vi "printScreen.vi"(8 "错误输出":errorcluster, 10 "记录时间":string, 11 "地址":refnum<visa-resource-name>) -> (0 "error out":errorcluster, 1 "图片路径":string, 3 "二维图片":picture)   [LabVIEW 2014]
panel:
  in  "路径":path=path "C:/image"
  in  "User name":string="anonymous"
  in  "Password":string="\n"
  out "standard output":string
  out "standard error":string
  in  "run minimized? (F)":bool=TRUE
  in  "path to BMP file":path=path "C:/image/gwt.png" caption="文件路径"
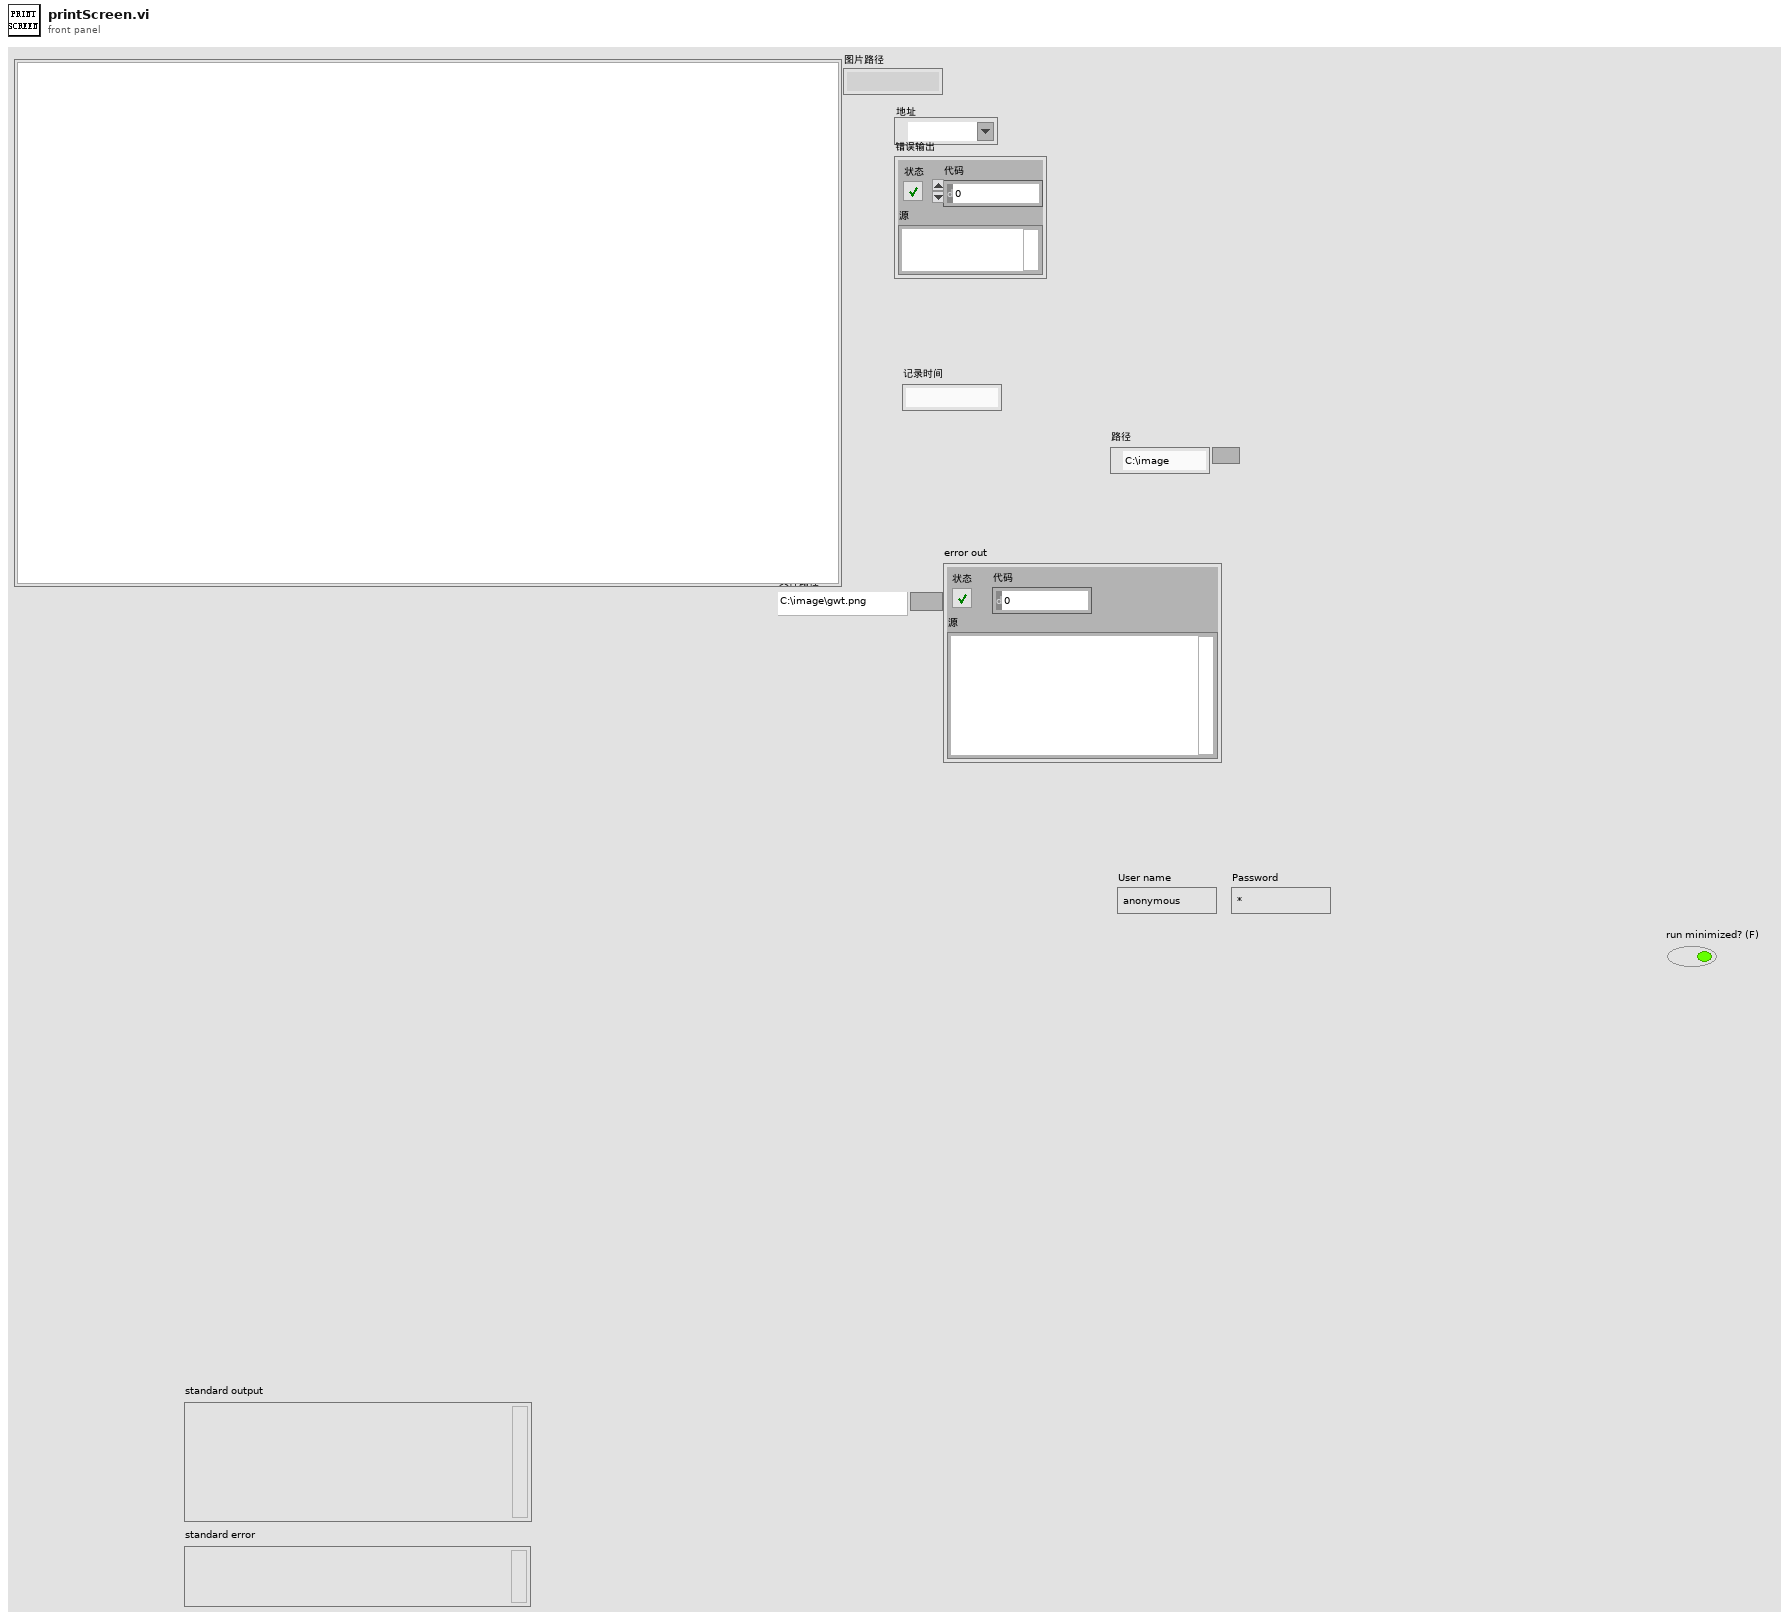
[diagram p1: front panel]
types:
  T1 = typedef "imagedata.ctl" = cluster{"image type":i32, "image depth":i32, "image":u8[], "mask":u8[], "colors":u32[], "Rectangle":cluster{"left":i16, "top":i16, "right":i16, "bottom":i16}}
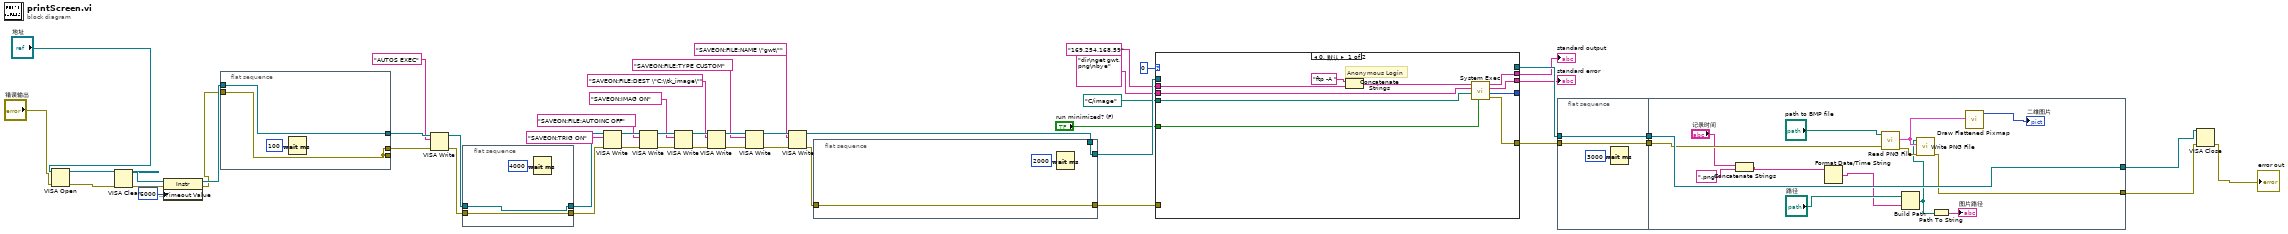
[diagram p0: block diagram]
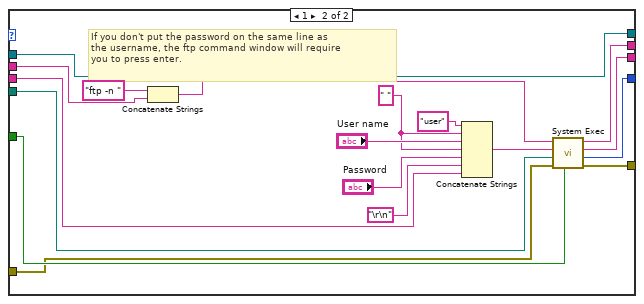
[diagram p2: hidden frame]
diagram:
  n1 = VISA Open(error in (no error)="错误输出", VISA resource name="地址") -> (VISA resource name=w9:refnum<visa-resource-name>, error out=w10:errorcluster)  [unwired: 3 in]
  n2 = VISA Clear(VISA resource name=w9, error in (no error)=w10) -> (VISA resource name out=w11:refnum<visa-resource-name>, error out=w12:errorcluster)
  n3 = property class="Instr"(reference=w11, error in=w12, "General Settings:Timeout Value"=u32 6000) -> (reference out=w5:refnum<visa-resource-name>, error out=w4:errorcluster)
  n4 = flat-sequence {
    tunnel: w5 -> [w53]
    tunnel: [w53] -> w47
    tunnel: [w52] -> _
    tunnel: w4 -> [w52]
    tunnel: [w52] -> w48
    frame #0 {
      n5 = Wait (ms)(milliseconds to wait=u32 100 ("等待时间（毫秒）")) -> ()  [unwired: 1 out]
    }
  }
  n6 = VISA Write(VISA resource name=w47, write buffer="AUTOS EXEC" ("写入缓冲区"), error in (no error)=w48) -> (VISA resource name out=w36:refnum<visa-resource-name>, error out=w37:errorcluster)  [unwired: 1 out]
  n7 = flat-sequence {
    tunnel: w36 -> [w55]
    tunnel: [w55] -> w39
    tunnel: w37 -> [w54]
    tunnel: [w54] -> w38
    frame #0 {
      n8 = Wait (ms)(milliseconds to wait=u32 4000 ("等待时间（毫秒）")) -> ()  [unwired: 1 out]
    }
  }
  n9 = VISA Write(VISA resource name=w39, write buffer="SAVEON:TRIG ON", error in (no error)=w38) -> (VISA resource name out=w25:refnum<visa-resource-name>, error out=w26:errorcluster)  [unwired: 1 out]
  n10 = VISA Write(VISA resource name=w25, write buffer="SAVEON:FILE:AUTOINC OFF" ("写入缓冲区"), error in (no error)=w26) -> (VISA resource name out=w27:refnum<visa-resource-name>, error out=w28:errorcluster)  [unwired: 1 out]
  n11 = VISA Write(VISA resource name=w27, write buffer="SAVEON:IMAG ON", error in (no error)=w28) -> (VISA resource name out=w21:refnum<visa-resource-name>, error out=w20:errorcluster)  [unwired: 1 out]
  n12 = VISA Write(VISA resource name=w21, write buffer="SAVEON:FILE:DEST \"C:\\tk_image\"" ("写入缓冲区"), error in (no error)=w20) -> (VISA resource name out=w23:refnum<visa-resource-name>, error out=w24:errorcluster)  [unwired: 1 out]
  n13 = VISA Write(VISA resource name=w23, write buffer="SAVEON:FILE:TYPE CUSTOM" ("写入缓冲区"), error in (no error)=w24) -> (VISA resource name out=w18:refnum<visa-resource-name>, error out=w19:errorcluster)  [unwired: 1 out]
  n14 = VISA Write(VISA resource name=w18, write buffer="SAVEON:FILE:NAME \"gwt\"" ("写入缓冲区"), error in (no error)=w19) -> (VISA resource name out=w43:refnum<visa-resource-name>, error out=w41:errorcluster)  [unwired: 1 out]
  n15 = flat-sequence {
    tunnel: [w59] -> w42
    tunnel: w43 -> [w57]
    tunnel: [w57] -> w44
    tunnel: w41 -> [w59]
    frame #0 {
      n16 = Wait (ms)(milliseconds to wait=u32 2000 ("等待时间（毫秒）")) -> ()  [unwired: 1 out]
    }
  }
  n17 = case shown="0, 默认" u16 0 ("Ring") {
    tunnel: [w65 w87] -> w29
    tunnel: [w69 w86] -> w30
    tunnel: [w68 w85] -> _
    tunnel: [w67 w84] -> w45
    tunnel: "run minimized? (F)" -> [w66 w83]
    tunnel: "169.254.168.59" -> [w64 w82]
    tunnel: path "C:/image" -> [w61 w79]
    tunnel: "dir\nget gwt.png\nbye" -> [w60 w76]
    tunnel: w42 -> [_ w71]
    tunnel: w44 -> [_ w70]
    tunnel: [_ w70] -> w46
    frame 0, Default {
      # "Anonymous Login"
      n18 = Concatenate Strings("ftp -A ", w64) -> (w63:string)
      n19 = call <vilib>:"System Exec.vi"("run minimized? (F)"=w66, "working directory"=w61, "standard input"=w60, "command line"=w63) -> ("error out"=w67:errorcluster, "return code"=w68:i32, "standard error"=w69:string, "standard output"=w65:string)  [unwired: 4 in]
    }
    frame 1 {
      w74 = " "
      # "If you don't put the password on the same line as\nthe username, the ftp command window will require \nyou to press enter."
      n20 = Concatenate Strings("ftp -n " ("command line"), w82) -> (w80:string)
      n21 = Concatenate Strings("user", w74, "User name", w74, "Password", "\r\n", w76) -> (w72:string)
      n22 = call <vilib>:"System Exec.vi"("run minimized? (F)"=w83, "error in (no error)"=w71, "working directory"=w79, "standard input"=w72, "command line"=w80) -> ("error out"=w84:errorcluster, "return code"=w85:i32, "standard error"=w86:string, "standard output"=w87:string)  [unwired: 3 in]
    }
  }
  "standard output" <- w29
  "standard error" <- w30
  n23 = flat-sequence {
    tunnel: w45 -> [w90]
    tunnel: [w90] -> w50
    tunnel: w46 -> [w89]
    tunnel: [w89] -> w49
    tunnel: [w104] -> w3
    tunnel: w49 -> [w104]
    tunnel: w50 -> [w101]
    tunnel: [w100] -> w2
    frame #0 {
      n24 = Wait (ms)(milliseconds to wait=u32 3000 ("等待时间（毫秒）")) -> ()  [unwired: 1 out]
    }
    frame #1 {
      n25 = Concatenate Strings("记录时间", ".png" ("时间格式字符串(%c)")) -> (w93:string)
      n26 = Format Date/Time String(time format string (%c)=w93) -> (date/time string=w98:string)  [unwired: 2 in]
      n27 = call <vilib>:"Read PNG File.vi"("error in (no error)"=w101, "path to PNG file"="path to BMP file") -> ("error out"=w102:errorcluster, "image data"=w97:T1)  [unwired: 7 in, 1 out]
      n28 = Build Path(base path="路径", name or relative path=w98) -> (appended path=w92:path)
      n29 = call <vilib>:"Write PNG File.vi"("error in (no error)"=w102, "image data"=w97, "path to PNG file"=w92) -> ("error out"=w100:errorcluster)  [unwired: 7 in, 1 out]
      n30 = Path To String(path=w92) -> (string=→"图片路径":string)
      n31 = call <vilib>:"Draw Flattened Pixmap.vi"("image data"=w97) -> ("new picture"=→"二维图片":picture)  [unwired: 8 in]
    }
  }
  n32 = VISA Close(VISA resource name=w3, error in (no error)=w2) -> (error out=→"error out":errorcluster)
